vi "Set RTB Selection Text Color.vi"(8 "Error In":errorcluster, 9 "Text Color":T1=enum."Black", 11 ".NET RTB Refnum in":refnum<k24>) -> (0 "Error Out":errorcluster, 3 ".NET RTB Refnum out":refnum<k24>)   [LabVIEW 2021, in "Rich Text Box.lvlib"]
uses:
  Rich Text Box.lvlib
  Text Colors.ctl
  System.Windows.Forms
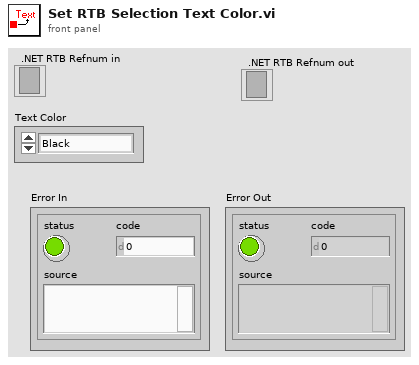
[diagram p1: front panel]
types:
  T1 = typedef "Rich Text Box.lvlib/Text Colors.ctl" = enum16{"Unchanged", "Black", "Blue", "Cyan", "Maroon", "Gray", "Violet", "Green", "Light Green", "Orange", "Yellow", "Magenta", "Red", "White"}
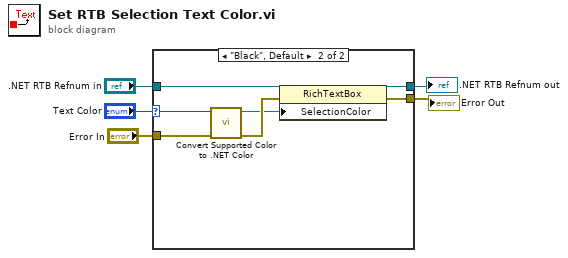
[diagram p0: block diagram]
diagram:
  n1 = case shown="\"Black\", Default" "Text Color" {
    selector: "Text Color" -> [_ w11]
    tunnel: ".NET RTB Refnum in" -> [w7 w12]
    tunnel: [w7 w10] -> w3
    tunnel: [w6 w9] -> w2
    tunnel: "Error In" -> [w6 w8]
    frame "Unchanged" {
    }
    frame "Black", Default {
      n2 = call "Convert Supported Color to .NET Color.vi"("error in (no error)"=w8, "Text Color"=w11) -> ("error out"=w14:errorcluster, ".NET Color"=w13:refnum<k24>)  [unwired: 8 in]
      n3 = property class="RichTextBox"(reference=w12, error in=w14, "SelectionColor"=w13) -> (reference out=w10:refnum<k24>, error out=w9:errorcluster)
    }
  }
  ".NET RTB Refnum out" <- w3
  "Error Out" <- w2
